vi "ElevatorBase_SLND.vi"(8 "CargoPick":bool, 9 "CargoDeliv":bool, 10 "Carry":bool, 11 "Hatch":bool) -> ()   [LabVIEW 2018]
uses:
  <vilib>/Rock Robotics/WPI/Solenoid/Deprecated/WPI_SolenoidSetBool.vi
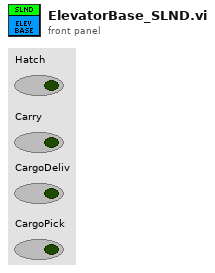
[diagram p1: front panel]
types:
  T1 = typedef "WPI_SolenoidDevRef.ctl" = cluster{"DevStatus":errorcluster, "Pneumatics Control Module":u8, "Forward Solenoid Channel":T2, "Reverse Solenoid Channel":T2}
  T2 = typedef "WPI_SolenoidChannel.ctl" = enum8{"Solenoid 0", "Solenoid 1", "Solenoid 2", "Solenoid 3", "Solenoid 4", "Solenoid 5", "Solenoid 6", "Solenoid 7", "Invalid"}
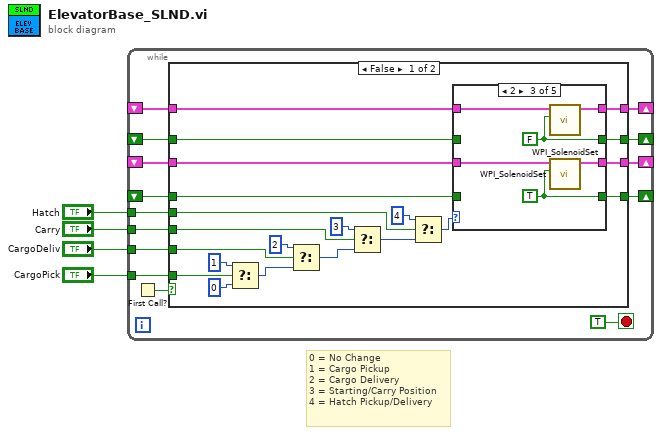
[diagram p0: block diagram]
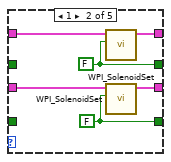
[diagram p3: hidden frame]
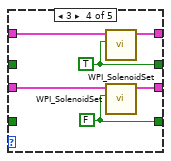
[diagram p4: hidden frame]
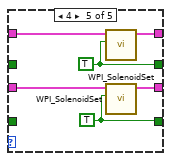
[diagram p5: hidden frame]
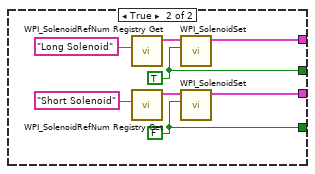
[diagram p6: hidden frame]
diagram:
  # "0 = No Change\n1 = Cargo Pickup\n2 = Cargo Delivery\n3 = Starting/Carry Position\n4 = Hatch Pickup/Delivery"
  n1 = while {
    tunnel: "CargoPick" -> [w17]
    tunnel: "CargoDeliv" -> [w16]
    tunnel: "Carry" -> [w15]
    tunnel: "Hatch" -> [w14]
    shift-right: [w13] -> _
    shift-left: _ -> [w11]
    shift-right: [w12] -> _
    shift-left: _ -> [w10]
    shift-right: [w9] -> _
    shift-left: _ -> [w7]
    shift-right: [w8] -> _
    shift-left: _ -> [w6]
    stop <- TRUE stop-if-true
    n2 = First Call?() -> (First Call?: T/F=w5:bool)
    n3 = case shown="False" w5 {
      tunnel: w17 -> [w35 _]
      tunnel: w16 -> [w34 _]
      tunnel: w15 -> [w33 _]
      tunnel: w14 -> [w32 _]
      tunnel: [w26 w72] -> w13
      tunnel: [w25 w73] -> w12
      tunnel: w11 -> [w24 _]
      tunnel: w10 -> [w23 _]
      tunnel: [w21 w69] -> w9
      tunnel: [w19 w68] -> w8
      tunnel: w7 -> [w22 _]
      tunnel: w6 -> [w20 _]
      frame False {
        n4 = Select(t=1, s=w35, f=0) -> (s? t:f=w38:i32)
        n5 = Select(t=2, s=w34, f=w38) -> (s? t:f=w37:i32)
        n6 = Select(t=3, s=w33, f=w37) -> (s? t:f=w36:i32)
        n7 = Select(t=4, s=w32, f=w36) -> (s? t:f=w27:i32)
        n8 = case shown="2" w27 {
          tunnel: [w43 w49 w55 w61 w67] -> w26
          tunnel: [w42 w48 w54 w60 w66] -> w25
          tunnel: w24 -> [w43 w47 w53 w59 w65]
          tunnel: w23 -> [w42 w46 w52 w58 w64]
          tunnel: w22 -> [w41 _ _ _ _]
          tunnel: [w41 w44 w51 w57 w62] -> w21
          tunnel: w20 -> [w40 _ _ _ _]
          tunnel: [w40 w45 w50 w56 w63] -> w19
          frame 0, Default {
          }
          frame 1 {
            w45 = FALSE
            w44 = FALSE
            n9 = call-poly <vilib>:"WPI_SolenoidSet.vi"("Value"=w45, "SolenoidDevRef"=w46) -> ("SolenoidDevRef"=w48:T1)  [unwired: 8 in, 1 out]
            n10 = call-poly <vilib>:"WPI_SolenoidSet.vi"("Value"=w44, "SolenoidDevRef"=w47) -> ("SolenoidDevRef"=w49:T1)  [unwired: 8 in, 1 out]
          }
          frame 2 {
            w50 = FALSE
            w51 = TRUE
            n11 = call-poly <vilib>:"WPI_SolenoidSet.vi"("Value"=w50, "SolenoidDevRef"=w52) -> ("SolenoidDevRef"=w54:T1)  [unwired: 8 in, 1 out]
            n12 = call-poly <vilib>:"WPI_SolenoidSet.vi"("Value"=w51, "SolenoidDevRef"=w53) -> ("SolenoidDevRef"=w55:T1)  [unwired: 8 in, 1 out]
          }
          frame 3 {
            w56 = TRUE
            w57 = FALSE
            n13 = call-poly <vilib>:"WPI_SolenoidSet.vi"("Value"=w56, "SolenoidDevRef"=w58) -> ("SolenoidDevRef"=w60:T1)  [unwired: 8 in, 1 out]
            n14 = call-poly <vilib>:"WPI_SolenoidSet.vi"("Value"=w57, "SolenoidDevRef"=w59) -> ("SolenoidDevRef"=w61:T1)  [unwired: 8 in, 1 out]
          }
          frame 4 {
            w63 = TRUE
            w62 = TRUE
            n15 = call-poly <vilib>:"WPI_SolenoidSet.vi"("Value"=w63, "SolenoidDevRef"=w64) -> ("SolenoidDevRef"=w66:T1)  [unwired: 8 in, 1 out]
            n16 = call-poly <vilib>:"WPI_SolenoidSet.vi"("Value"=w62, "SolenoidDevRef"=w65) -> ("SolenoidDevRef"=w67:T1)  [unwired: 8 in, 1 out]
          }
        }
      }
      frame True {
        w68 = TRUE
        w69 = FALSE
        n17 = call <vilib>:"WPI_SolenoidRefNum Registry Get.vi"("refnum name"="Long Solenoid") -> ("SolenoidDevRef"=w70:T1)  [unwired: 9 in, 1 out]
        n18 = call <vilib>:"WPI_SolenoidRefNum Registry Get.vi"("refnum name"="Short Solenoid") -> ("SolenoidDevRef"=w71:T1)  [unwired: 9 in, 1 out]
        n19 = call-poly <vilib>:"WPI_SolenoidSet.vi"("Value"=w68, "SolenoidDevRef"=w70) -> ("SolenoidDevRef"=w73:T1)  [unwired: 8 in, 1 out]
        n20 = call-poly <vilib>:"WPI_SolenoidSet.vi"("Value"=w69, "SolenoidDevRef"=w71) -> ("SolenoidDevRef"=w72:T1)  [unwired: 8 in, 1 out]
      }
    }
  }
